vi "addFoodInfo.vi"(5 "error in (no error)":errorcluster caption="错误输入（无错误）", 8 "食品信息":cluster{"ID":dbl, "食品名称":string, "价格":dbl}, 9 "数组":cluster{"ID":dbl, "食品名称":string, "价格":dbl}[](array[cluster])) -> (4 "error out":errorcluster caption="错误输出")   [LabVIEW 2013, in "FoodBase.lvclass"]
doc: "该模板用于创建子VI。"
uses:
  FoodBase.lvclass
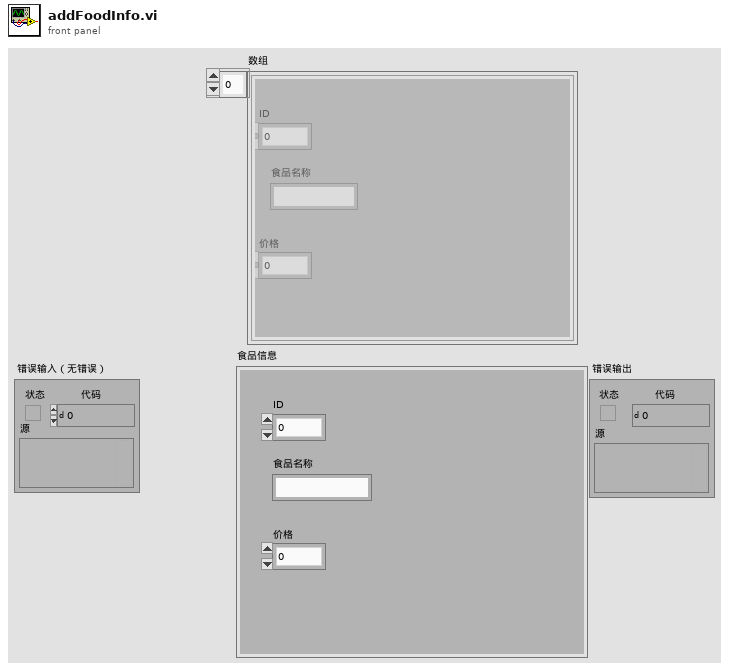
[diagram p1: front panel]
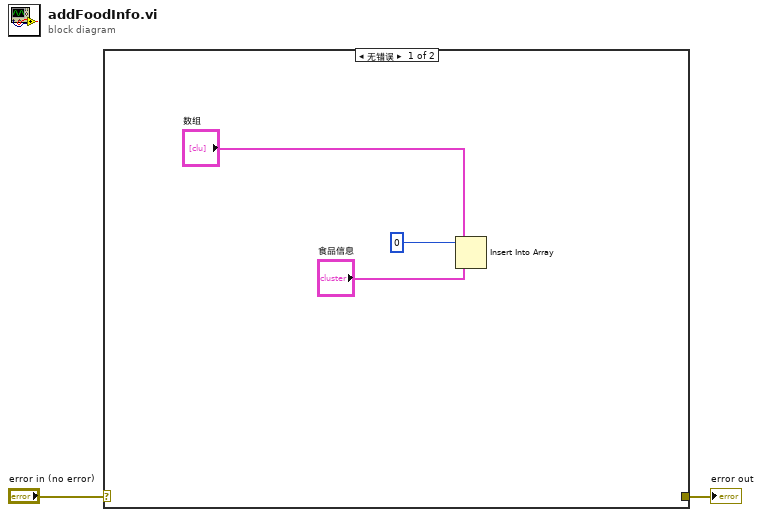
[diagram p0: block diagram]
diagram:
  n1 = case shown="无错误" "error in (no error)" {
    selector: "error in (no error)" -> [_ w6]
    tunnel: [_ w6] -> w1
    frame No Error {
      n2 = Insert Into Array(array="数组", index=0, new element="食品信息") -> ()  [unwired: 1 out]
    }
    frame Error {
    }
  }
  "error out" <- w1
